vi "Internal Power Supply Test.vi"(5 "Device":string, 9 "Delay Time (s)":dbl=0.1, 10 "input terminal configuration":i32(ring)=10078 items=["default"=-1, "RSE"=10083, "NRSE"=10078, "Differential"=10106, "Pseudodifferential"=12529], 11 "Voltage Selector":T1=enum."+3.3V") -> (0 "error out":errorcluster, 3 "Voltage":dbl format="%.4f")   [LabVIEW 2015]
uses:
  DAQ/Internal Voltages.ctl
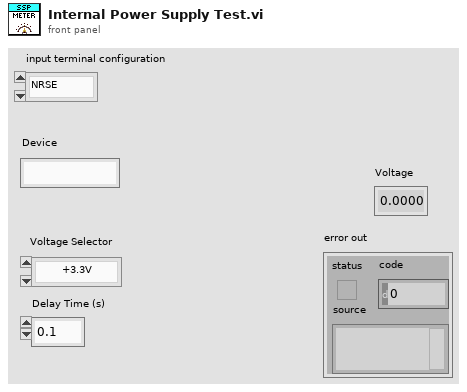
[diagram p1: front panel]
types:
  T1 = typedef "Internal Voltages.ctl" = enum16{"REF-2.5", "+3.3V", "+5.2V", "+5.2VA", "-5.2VA", "+1.6V", "NONE"}
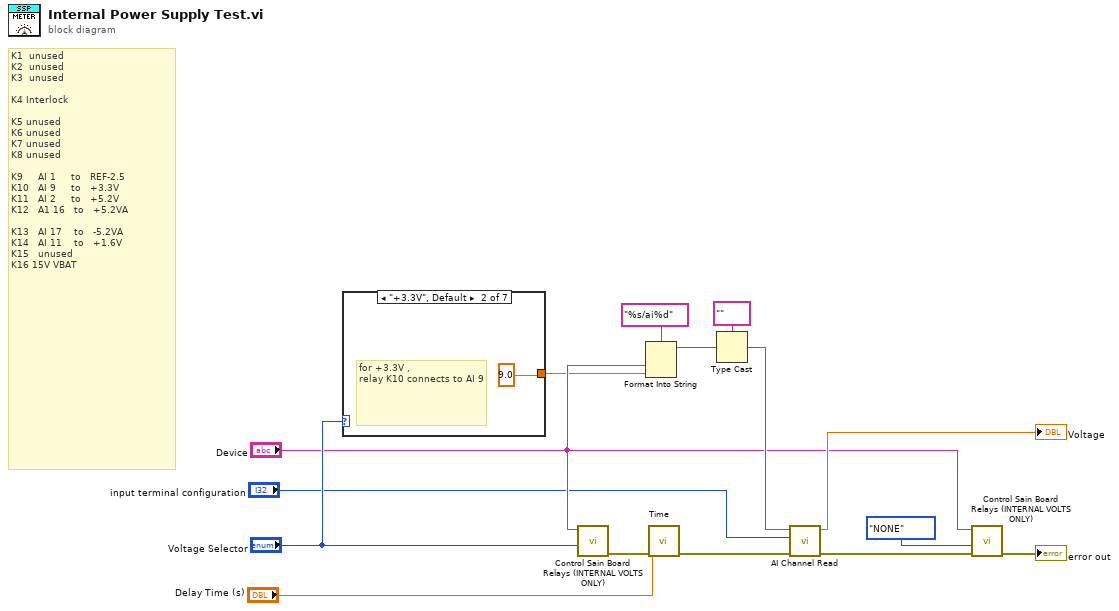
[diagram p0: block diagram]
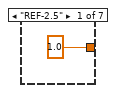
[diagram p2: hidden frame]
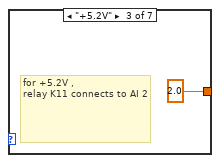
[diagram p3: hidden frame]
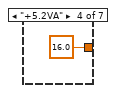
[diagram p4: hidden frame]
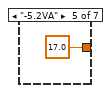
[diagram p5: hidden frame]
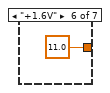
[diagram p6: hidden frame]
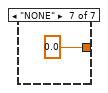
[diagram p7: hidden frame]
diagram:
  # "K1  unused \nK2  unused\nK3  unused\n\nK4 Interlock\n\nK5 unused\nK6 unused\nK7 unused\nK8 unused\n\nK9     AI 1     to   REF-2.5\nK10   AI 9     to   +3.3V\nK11   AI 2     to   +5.2V\nK12   A1 16   to   +5.2VA\n\nK13   AI 17    to   -5.2VA\nK14   AI 11    to   +1.6V\nK15   unused \nK16 15V VBAT"
  n1 = case shown="\"+3.3V\", Default" "Voltage Selector" {
    tunnel: [1.0 9.0 2.0 16.0 17.0 11.0 0.0] -> w2
    frame "REF-2.5" {
    }
    frame "+3.3V", Default {
      # "for +3.3V , \nrelay K10 connects to AI 9"
    }
    frame "+5.2V" {
      # "for +5.2V , \nrelay K11 connects to AI 2"
    }
    frame "+5.2VA" {
    }
    frame "-5.2VA" {
    }
    frame "+1.6V" {
    }
    frame "NONE" {
    }
  }
  n2 = call "Control Sain Board Relays (INTERNAL VOLTS ONLY).vi"("Voltage"="Voltage Selector", "Device Name"="Device") -> ("error out"=w14:errorcluster)  [unwired: 9 in]
  n3 = Format Into String(format string="%s/ai%d", "Device", w2) -> (resulting string=w4:string)  [unwired: 2 in, 1 out]
  n4 = call "Time"("error in (no error)"=w14, "Delay Time (s)"="Delay Time (s)") -> ("error out"=w9:errorcluster)  [unwired: 9 in]
  n5 = Type Cast(type=tag "" ("lines"), x=w4) -> (*(type *) &x=w6:tag)
  n6 = call "AI Channel Read.vi"("error in"=w9, "input terminal configuration"="input terminal configuration", "physical channels"=w6) -> ("error out"=w13:errorcluster, "data"=→"Voltage":dbl)  [unwired: 7 in]
  n7 = call "Control Sain Board Relays (INTERNAL VOLTS ONLY).vi"("error in"=w13, "Voltage"=Internal_Voltages."NONE", "Device Name"="Device") -> ("error out"=→"error out":errorcluster)  [unwired: 8 in]
